vi "fpga_read_data.vi"(6 "Scaler":dbl=1.0, 8 "error in":errorcluster, 9 "Timeout (ms)":i32=5000, 10 "Number of Elements":u32, 11 "FPGA VI Reference in":T2) -> (0 "error out":errorcluster, 1 "Elements remaining":T1, 2 "Raw_streams_array":dbl[][](array[numeric]), 3 "FPGA VI Reference Out":T2)   [LabVIEW 2011, in "Fiberscope_library.lvlib"]
uses:
  Fiberscope_library.lvlib
  typedefs/fpga_main_spiral_fpga_ref.ctl
  <vilib>/Utility/error.llb/Error Cluster From Error Code.vi
  <vilib>/rvi/errors/niLvFpgaAdjustHostInterfaceError.vi
  <vilib>/rvi/interface/nirviMethod/nirviMethod.xnode
  FPGA Bitfiles/FiberscopeRK1107_FPGATarget_fpgamainspiral_0DF2A7CB.lvbitx
  <vilib>/FPGAPlugInAG/PXI-7813R/niLvFpga_ReadFifo_PXI-7813R.vi
  <vilib>/rvi/errors/niLvFpgaMergeErrorWithErrorCode.vi
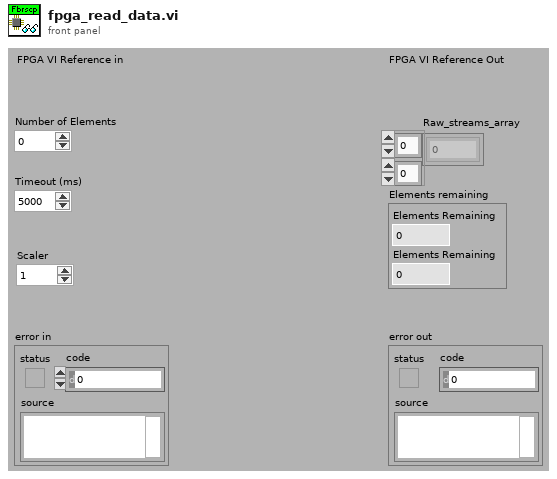
[diagram p1: front panel]
types:
  T1 = cluster{"Elements Remaining":u32, "Elements Remaining":u32}
  T2 = typedef "Fiberscope_library.lvlib/fpga_main_spiral_fpga_ref.ctl" = refnum<k20>
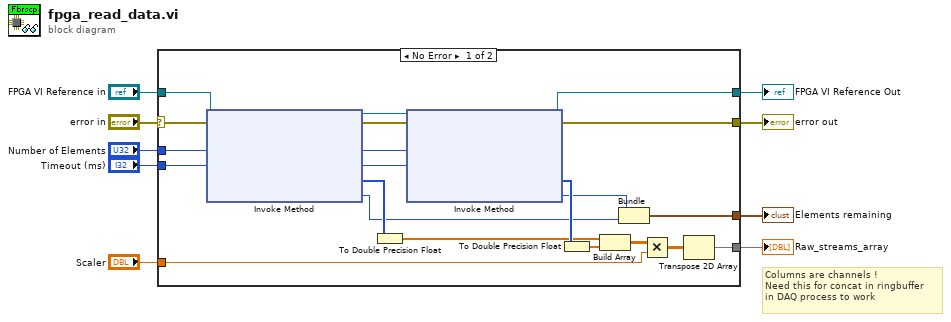
[diagram p0: block diagram]
diagram:
  # "Columns are channels !\nNeed this for concat in ringbuffer\nin DAQ process to work"
  n1 = case shown="No Error" "error in" {
    selector: "error in" -> [w28 w30]
    tunnel: [w24 w30] -> w8
    tunnel: "FPGA VI Reference in" -> [w27 w29]
    tunnel: [w23 w29] -> w6
    tunnel: "Number of Elements" -> [w22 _]
    tunnel: "Timeout (ms)" -> [w21 _]
    tunnel: [w17 _] -> w3
    tunnel: [w14 _] -> w2
    tunnel: "Scaler" -> [w10 _]
    frame No Error {
      n2 = xnode "Invoke Method"("FPGA VI Reference In"=w27, "error in"=w28, "Number of Elements"=w22, "Timeout (ms)"=w21) -> ("FPGA VI Reference Out"=w25:T2, "error out"=w26:errorcluster, "Data"=w20:u16[], "Elements Remaining"=w16:u32)
      n3 = To Double Precision Float(number=w20) -> (double precision float=w13:dbl[])
      n4 = xnode "Invoke Method"("FPGA VI Reference In"=w25, "error in"=w26, "Number of Elements"=w22, "Timeout (ms)"=w21) -> ("FPGA VI Reference Out"=w23:T2, "error out"=w24:errorcluster, "Data"=w19:u16[], "Elements Remaining"=w15:u32)
      n5 = To Double Precision Float(number=w19) -> (double precision float=w18:dbl[])
      n6 = Build Array(w13, w18) -> (w12:dbl[][])
      n7 = Bundle("Elements Remaining"=w15, "Elements Remaining"=w16) -> (w14:T1)  [unwired: 1 in]
      n8 = Multiply(x=w12, y=w10) -> (x*y=w11:dbl[][])
      n9 = Transpose 2D Array(2D array=w11) -> (transposed array=w17:dbl[][])
    }
    frame Error {
    }
  }
  "error out" <- w8
  "FPGA VI Reference Out" <- w6
  "Raw_streams_array" <- w3
  "Elements remaining" <- w2
